vi "Longitudinal Profile.vi"(5 "Long.X-Locations":dbl[](array[numeric])=[-500.0, -250.0, 0.0, 250.0, 500.0], 6 "Averaging time (min)":dbl, 7 "Lat.Coords":T1={"X"=-3390.0, "Y"=-113.0, "Z"=780.0, "Name"="Anemo1", "Spacing"=enum."Specified", "start"=780.0, "end"=780.0, "NumPts"=780.0, "Specified Locns"=[]}, 9 "Direction":enum16{"Forward", "Reverse"}(ring), 10 "Tunnel Speed":dbl, 11 "Input Task Array":T2[](array[typedef]) {"Carrier_2 Q (l/min)" format="%#.2f"; "Row Duration (mins)" format="%#.1f"; "Row No" min=0; "Trace Gas Concentration (%)" min=0.0 format="%#_4f"; "Carrier_1 Q (l/min)" format="%#.2f"; "Tunnel Speed" format="%#.2f"; "Start X" format="%#.2f"; "Start Y" format="%#.2f"; "Start Z" format="%#.2f"; "End X" format="%#.2f"; "End Y" format="%#.2f"; "End Z" format="%#.2f"; "Averaging time (min)" min=0.0 format="%#.2f"}) -> (3 "Output Task Array":T2[](array[typedef]) {"Carrier_2 Q (l/min)" format="%#.2f"; "Row Duration (mins)" format="%#.1f"; "Row No" min=0; "Trace Gas Concentration (%)" min=0.0 format="%#_4f"; "Carrier_1 Q (l/min)" format="%#.2f"; "Tunnel Speed" format="%#.2f"; "Start X" format="%#.2f"; "Start Y" format="%#.2f"; "Start Z" format="%#.2f"; "End X" format="%#.2f"; "End Y" format="%#.2f"; "End Z" format="%#.2f"; "Averaging time (min)" min=0.0 format="%#.2f"})   [LabVIEW 2016]
uses:
  RowTemplate.ctl
  Anemometry Sub Vis/Gen Trav/Spacing.ctl
  Anemometry Sub Vis/Controls/Multi_run_mode.ctl
  MRCMDFBGlobal.vi
panel:
  # "X           Y            Z"
  # "Start"
  # "End"
  # "X           Y            Z"
  # "Start"
  # "End"
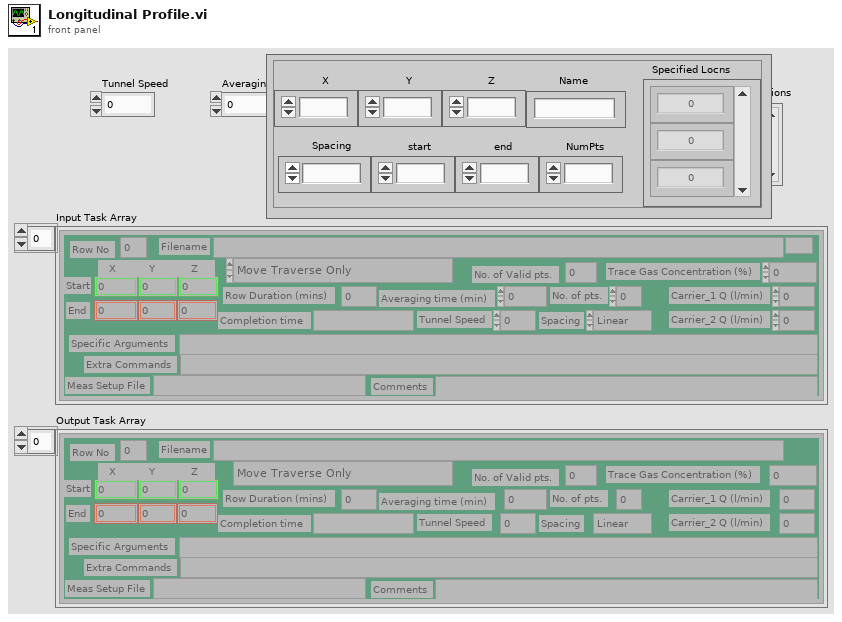
[diagram p1: front panel]
types:
  T1 = cluster{"X":dbl, "Y":dbl, "Z":dbl, "Name":string, "Spacing":enum16{"Linear", "Log", "Gauss", "Specified", "N/A"}, "start":dbl, "end":dbl, "NumPts":dbl, "Specified Locns":dbl[]}
  T2 = typedef "RowTemplate.ctl" = cluster{"Start X":sgl, "Start Y":sgl, "Start Z":sgl, "End X":sgl, "End Y":sgl, "End Z":sgl, "No. of pts.":i32, "Spacing":T3, "Filename":path, "Tunnel Speed":dbl, "Averaging time (min)":dbl, "Extra Commands":string, "Carrier_1 Q (l/min)":dbl, "Carrier_2 Q (l/min)":dbl, "Trace Gas Concentration (%)":dbl, "Specific Arguments":string, "Comments":string, "Row No":i32, "Row Type Selector":T4, "Completion time":string, "Row Duration (mins)":dbl, "No. of Valid pts.":i32, "Meas Setup File":string}
  T3 = typedef "Spacing.ctl" = enum16{"Linear", "Log", "Gauss", "Specified", "N/A"}
  T4 = typedef "Multi_run_mode.ctl" = enum16{"Move Traverse Only", "Set Tunnel Speed Only", "Set Source Only", "Set Measurement Conditions", "Single Measurement", "Vertical Profile", "Lateral Profile", "Longitudinal Profile", "Explore Volume", "Multi-Axis Profile", "Auto Calibrate", "Meas Fast FID Bkgnd", "Check Beam Power", "Scanning Valve Measurement", "Run VI Named:", "Set ADAM Ch", "Wait (minutes)", "Send Message", "Synchronize With:", "Fall Back to this Row", "Turn Off Row Repeating", "Blank Row", "Traverse 3D Volume"}
  T5 = cluster{"Start X":sgl, "Start Y":sgl, "Start Z":sgl, "End X":sgl, "End Y":sgl, "End Z":sgl, "No. of pts.":i32, "Spacing":T3, "Filename":path, "Tunnel Speed":dbl, "Averaging time (min)":dbl, "Extra Commands":string, "Carrier_1 Q (l/min)":dbl, "Carrier_2 Q (l/min)":dbl, "Trace Gas Concentration (%)":dbl, "Specific Arguments":string, "Comments":string, "Row No":i32, "Row Type Selector":T4, "Completion time":string, "Row Duration (mins)":dbl, "No. of Valid pts.":i32, "Meas Setup File":string}
  T6 = enum16{"Linear", "Log", "Gauss", "Specified", "N/A"}
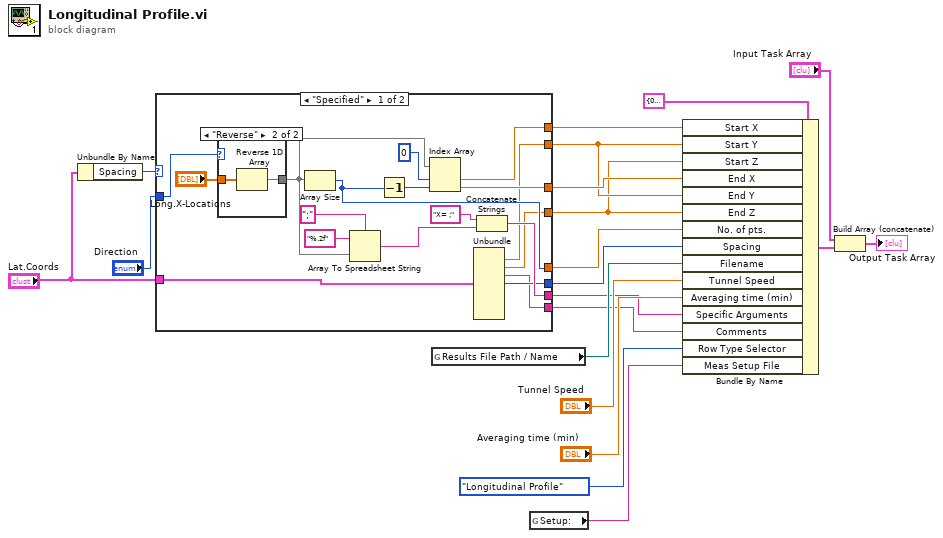
[diagram p0: block diagram]
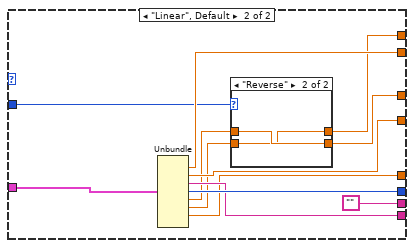
[diagram p3: hidden frame]
diagram:
  n1 = Unbundle By Name("Lat.Coords") -> ("Spacing"=w6:T6)
  n2 = case shown="\"Specified\"" w6 {
    tunnel: [w27 w52] -> w11
    tunnel: [w32 w47] -> w10
    tunnel: [w31 w42] -> w9
    tunnel: [w30 w43] -> w8
    tunnel: [w29 ""] -> w7
    tunnel: "Lat.Coords" -> [w28 w53]
    tunnel: [w26 w49] -> w5
    tunnel: [w25 w51] -> w4
    tunnel: [w24 w50] -> w3
    tunnel: "Direction" -> [w23 w46]
    frame "Specified" {
      n3 = case shown="\"Reverse\"" w23 {
        tunnel: "Long.X-Locations" -> [w39 w41]
        tunnel: [w39 w40] -> w21
        frame "Forward", Default {
        }
        frame "Reverse" {
          n4 = Reverse 1D Array(array=w41) -> (reversed array=w40:dbl[])
        }
      }
      n5 = Array Size(array=w21) -> (size(s)=w32:i32)
      n6 = Array To Spreadsheet String(delimiter (Tab)=";", array=w21, 3:"%.2f" ("format string")) -> (spreadsheet string=w34:string)
      n7 = Decrement(x=w32) -> (x-1=w35:i32)
      n8 = Index Array(array=w21, index #1=0 ("index"), index #2=w35) -> (element #1=w30:dbl, element #2=w31:dbl)
      n9 = Unbundle(w28) -> ("Y"=w25:dbl, "Z"=w24:dbl, "Name"=w26:string, "Spacing"=w27:T6)  [unwired: 5 out]
      n10 = Concatenate Strings("X= ;", w34) -> (w29:string)
    }
    frame "Linear", Default {
      n11 = Unbundle(w53) -> ("Y"=w51:dbl, "Z"=w50:dbl, "Name"=w49:string, "Spacing"=w52:T6, "start"=w45:dbl, "end"=w44:dbl, "NumPts"=w47:dbl)  [unwired: 2 out]
      n12 = case shown="\"Reverse\"" w46 {
        tunnel: w45 -> [w55 w57]
        tunnel: [w55 w56] -> w43
        tunnel: w44 -> [w54 w56]
        tunnel: [w54 w57] -> w42
        frame "Forward", Default {
        }
        frame "Reverse" {
        }
      }
    }
  }
  n13 = global read "MRCMDFBGlobal.vi" "Results File Path / Name"() -> (w12:path)
  n14 = global read "MRCMDFBGlobal.vi" "Setup:"() -> (w13:string)
  n15 = Bundle By Name(cluster=T5 {"Start X"=0.0, "Start Y"=0.0, "Start Z"=0.0, "End X"=0.0, "End Y"=0.0, "End Z"=0.0, "No. of pts."=0, "Spacing"=enum."Linear", "Filename"=path "", "Tunnel Speed"=0.0, "Averaging time (min)"=0.0, "Extra Commands"="", "Carrier_1 Q (l/min)"=0.0, "Carrier_2 Q (l/min)"=0.0, "Trace Gas Concentration (%)"=0.0, "Specific Arguments"="", "Comments"="", "Row No"=0, "Row Type Selector"=enum."Move Traverse Only", "Completion time"="", "Row Duration (mins)"=0.0, "No. of Valid pts."=0, "Meas Setup File"=""} ("RowTemplateConst"), "Start X"=w8, "Start Y"=w4, "Start Z"=w3, "End X"=w9, "End Y"=w4, "End Z"=w3, "No. of pts."=w10, "Spacing"=w11, "Filename"=w12, "Tunnel Speed"="Tunnel Speed", "Averaging time (min)"="Averaging time (min)", "Specific Arguments"=w7, "Comments"=w5, "Row Type Selector"=Multi_run_mode."Longitudinal Profile", "Meas Setup File"=w13) -> (w15:T5)
  n16 = Build Array (concatenate)("Input Task Array", w15) -> (→"Output Task Array":T2[])
